vi "UID.vi"(6 "Alias":string, 7 "Actor in":refnum<class "Actor.lvclass">) -> (0 "Error out":errorcluster, 2 "UID":i32)   [LabVIEW 2020, in "jettl.lvlib" / "Read Child Attributes.lvlib"]
uses:
  Read Child Attributes.lvlib
  jettl.lvlib
  Attributes/Attributes.lvclass
  Actor/Actor.lvclass
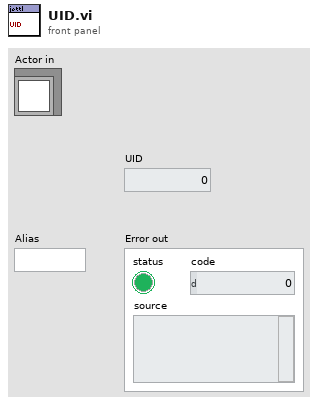
[diagram p1: front panel]
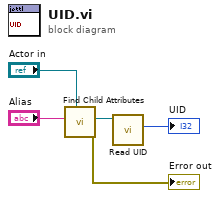
[diagram p0: block diagram]
diagram:
  n1 = call "Find Child Attributes.vi"("Actor in"="Actor in", "Alias"="Alias") -> ("Error out"=→"Error out":errorcluster, "Child Attributes"=w2:refnum<class "Attributes.lvclass">)  [unwired: 8 in]
  n2 = call-dynamic "Read UID.vi"("Attributes in"=w2) -> ("UID"=→"UID":i32)  [unwired: 10 in]
